vi "12-type_digital.vi"(2 "this":i32, 3 "button":i32, 4 "settings in":T2={"Auto1"=TRUE, "Auto2"=TRUE, "Rel1"=TRUE, "Rel2"=TRUE, "Filt1"=TRUE, "Filt2"=TRUE, "Rate"=enum."Med", "Range1"=enum."10mV", "Range2"=enum."100mV", "Filt3"=TRUE, "Filt4"=TRUE, "Rel temp"=TRUE, "Analog1"=FALSE, "Analog2"=FALSE, "Analog temp"=FALSE, "Digital1"=TRUE, "Digital2"=TRUE, "Digital temp "=TRUE, "Window1"=enum."0,01%", "Window2"=enum."0,01%", "Window temp"=enum."0,01%", "RDGS1"="010", "RDGS2"="010", "RDGS temp"="010", "Type_type1"=TRUE, "Type_type2"=TRUE, "Type_type temp"=TRUE, "LSync"=FALSE, "Unit"=enum."C", "Sens"=TRUE, "Type tcoupl"=enum."J", "Junc"=TRUE, "prevState"=0}) -> (0 "next state":i32, 1 "settings out":T1)   [LabVIEW 2017]
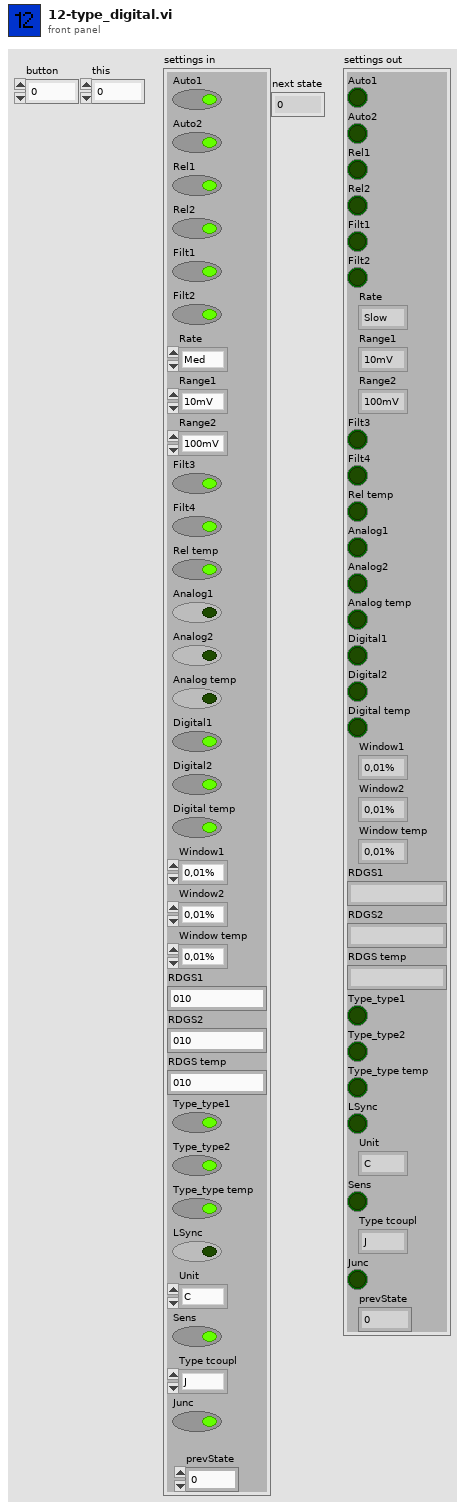
[diagram p1: front panel]
types:
  T1 = cluster{"Auto1":bool, "Auto2":bool, "Rel1":bool, "Rel2":bool, "Filt1":bool, "Filt2":bool, "Rate":enum16{"Slow", "Med", "Fast"}, "Range1":enum16{"10mV", "100mV", "1V", "10V", "100V"}, "Range2":enum16{"100mV", "1V", "10V"}, "Filt3":bool, "Filt4":bool, "Rel temp":bool, "Analog1":bool, "Analog2":bool, "Analog temp":bool, "Digital1":bool, "Digital2":bool, "Digital temp ":bool, "Window1":enum16{"0,01%", "0,1%", "1%", "10%", "None"}, "Window2":enum16{"0,01%", "0,1%", "1%", "10%", "None"}, "Window temp":enum16{"0,01%", "0,1%", "1%", "10%", "None"}, "RDGS1":string, "RDGS2":string, "RDGS temp":string, "Type_type1":bool, "Type_type2":bool, "Type_type temp":bool, "LSync":bool, "Unit":enum16{"C", "K", "F"}, "Sens":bool, "Type tcoupl":enum16{"J", "K", "T", "E", "R", "S", "B", "N"}, "Junc":bool, "prevState":dbl}
  T2 = cluster{"Auto1":bool, "Auto2":bool, "Rel1":bool, "Rel2":bool, "Filt1":bool, "Filt2":bool, "Rate":enum16{"Slow", "Med", "Fast"}, "Range1":enum16{"10mV", "100mV", "1V", "10V", "100V"}, "Range2":enum16{"100mV", "1V", "10V"}, "Filt3":bool, "Filt4":bool, "Rel temp":bool, "Analog1":bool, "Analog2":bool, "Analog temp":bool, "Digital1":bool, "Digital2":bool, "Digital temp ":bool, "Window1":enum16{"0,01%", "0,1%", "1%", "10%", "None"}, "Window2":enum16{"0,01%", "0,1%", "1%", "10%", "None"}, "Window temp":enum16{"0,01%", "0,1%", "1%", "10%", "None"}, "RDGS1":string, "RDGS2":string, "RDGS temp":string, "Type_type1":bool, "Type_type2":bool, "Type_type temp":bool, "LSync":bool, "Unit":enum16{"C", "K", "F"}, "Sens":bool, "Type tcoupl":enum16{"J", "K", "T", "E", "R", "S", "B", "N"}, "Junc":bool, "prevState":i32}
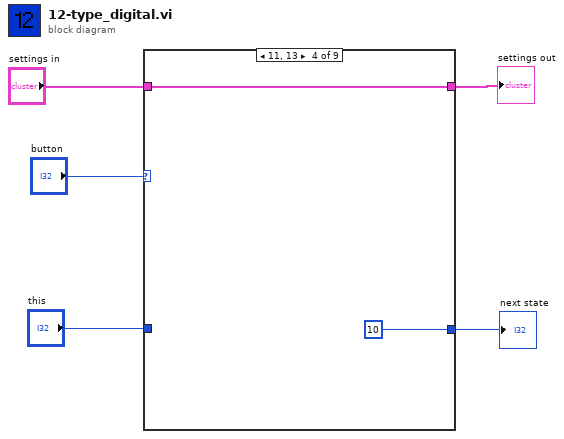
[diagram p0: block diagram]
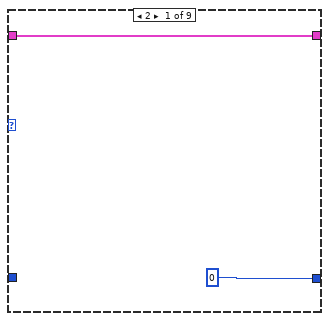
[diagram p2: hidden frame]
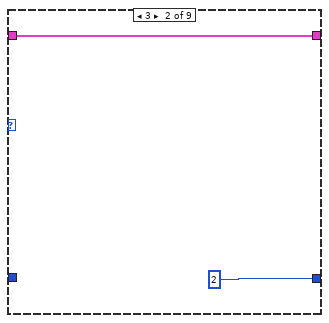
[diagram p3: hidden frame]
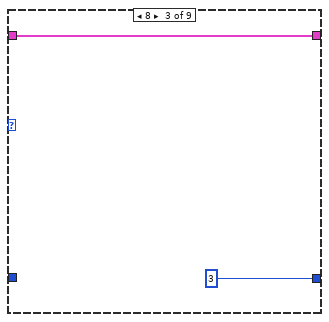
[diagram p4: hidden frame]
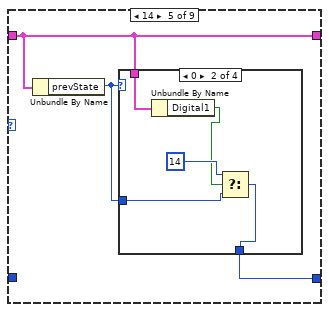
[diagram p5: hidden frame]
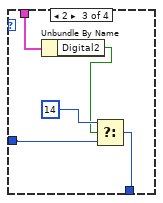
[diagram p7: hidden frame]
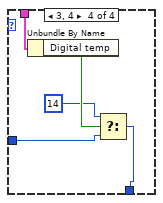
[diagram p8: hidden frame]
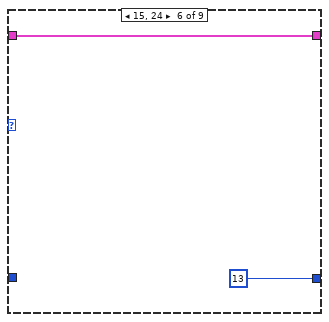
[diagram p9: hidden frame]
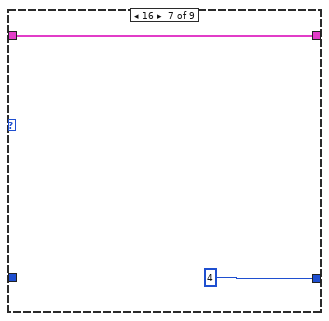
[diagram p10: hidden frame]
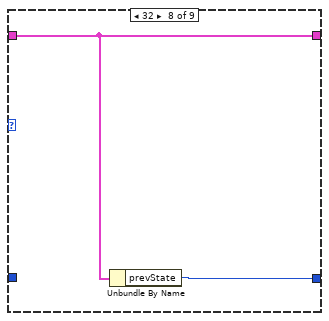
[diagram p11: hidden frame]
diagram:
  n1 = case shown="11, 13" "button" {
    tunnel: [0 ("this") 2 3 10 ("this") w15 13 ("this") 4 w37 w39] -> w2
    tunnel: "this" -> [_ _ _ _ _ _ _ _ w39]
    tunnel: "settings in" -> [w7 w8 w10 w13 w16 w34 w35 w38 w40]
    tunnel: [w7 w8 w10 w13 w16 w34 w35 w38 w40] -> w1
    frame 2 {
    }
    frame 3 {
    }
    frame 8 {
    }
    frame 11, 13 {
    }
    frame 14 {
      n2 = Unbundle By Name(w16) -> ("prevState"=w14:i32)
      n3 = case shown="0" w14 {
        tunnel: w16 -> [_ w22 w27 w32]
        tunnel: [w17 w18 w25 w28] -> w15
        tunnel: w14 -> [w17 w19 w24 w29]
        frame Default {
        }
        frame 0 {
          n4 = Unbundle By Name(w22) -> ("Digital1"=w20:bool)
          n5 = Select(t=14, s=w20, f=w19) -> (s? t:f=w18:i32)
        }
        frame 2 {
          n6 = Unbundle By Name(w27) -> ("Digital2"=w23:bool)
          n7 = Select(t=14, s=w23, f=w24) -> (s? t:f=w25:i32)
        }
        frame 3, 4 {
          n8 = Unbundle By Name(w32) -> ("Digital temp"=w31:bool)
          n9 = Select(t=14, s=w31, f=w29) -> (s? t:f=w28:i32)
        }
      }
    }
    frame 15, 24 {
    }
    frame 16 {
    }
    frame 32 {
      n10 = Unbundle By Name(w38) -> ("prevState"=w37:i32)
    }
    frame Default {
    }
  }
  "next state" <- w2
  "settings out" <- w1
